vi "Assignment_2_Boolean.vi"() -> ()   [LabVIEW 2019]
uses:
  <vilib>/numeric/Random Number (Range) U64.vi
  <vilib>/numeric/sub_Random U32.vi
panel:
  in  "y":bool
  in  "y":bool
  in  "lower bound (0)":u64
  in  "upper bound (100)":u64=100
  out "Random Number":u64
  out "0, 1":i16
  in  "Boolean":bool
  in  "value 5":dbl
  in  "value 4":dbl
  in  "value 3":dbl
  in  "value 2":dbl
  in  "value 1":dbl
  out "Result":i32
  out "Result":bool
  in  "y":bool
  in  "x":bool
  in  "T/F":bool
  out "Result":bool
  out "Result":bool
  in  "x":bool
  out "Result":bool
  in  "y":bool
  in  "x":bool
  out "Result":bool
  in  "x":bool
  # "Diagram Disabled Structure is used"
  # "And gate/Or gate"
  # "Not And gate/Not Or gate"
  # "Exclusive Or gate/Not Exclusive Or gate"
  # "Not gate"
  # "Implies Operator"
  # "Compond Arithmetic"
  # "Bool to (0, 1)"
  # "Random Number Generator"
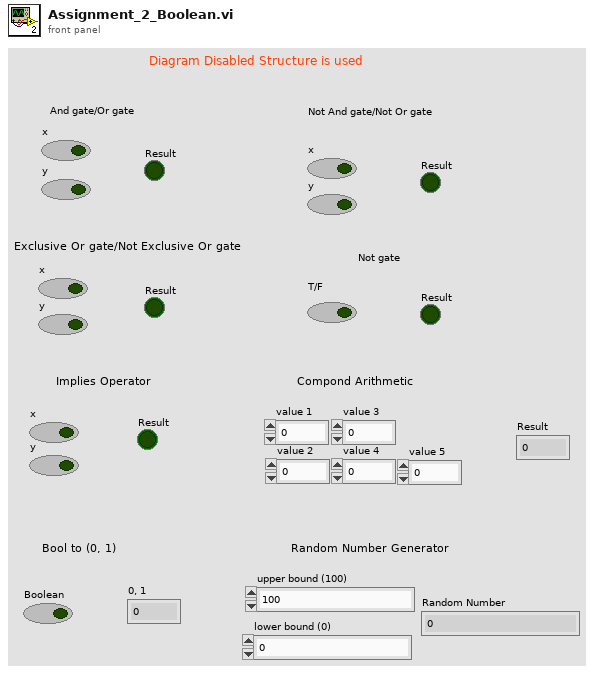
[diagram p1: front panel]
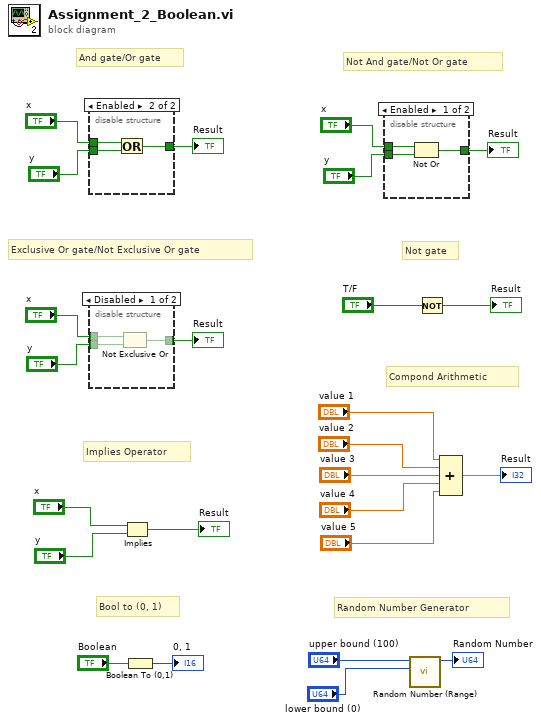
[diagram p0: block diagram]
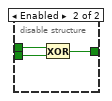
[diagram p2: hidden frame]
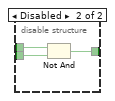
[diagram p3: hidden frame]
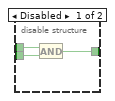
[diagram p4: hidden frame]
diagram:
  # "Random Number Generator"
  # "Bool to (0, 1)"
  # "Compond Arithmetic"
  # "Implies Operator"
  # "Not gate"
  # "Exclusive Or gate/Not Exclusive Or gate"
  # "Not And gate/Not Or gate"
  # "And gate/Or gate"
  n1 = disable-structure shown="Enabled" {
    disable-tunnel: "x" -> [w28 w30]
    disable-tunnel: "y" -> [w27 w29]
    disable-tunnel: [w26 w31] -> w24
    frame Disabled {
      n2 = And(x=w28, y=w27) -> (x .and. y?=w26:bool)
    }
    frame Enabled {
      n3 = Or(x=w30, y=w29) -> (x .or. y?=w31:bool)
    }
  }
  "Result" <- w24
  n4 = disable-structure shown="Disabled" {
    disable-tunnel: "x" -> [w33 w36]
    disable-tunnel: "y" -> [w32 w35]
    disable-tunnel: [w34 w37] -> w19
    frame Disabled {
      n5 = Not Exclusive Or(1:w32, 2:w33) -> (0:w34:bool)
    }
    frame Enabled {
      n6 = Exclusive Or(1:w35, 2:w36) -> (0:w37:bool)
    }
  }
  "Result" <- w19
  n7 = Implies(1:"y", 2:"x") -> (0:→"Result":bool)
  n8 = Boolean To (0,1)(Boolean="Boolean") -> (0, 1=→"0, 1":i16)
  n9 = disable-structure shown="Enabled" {
    disable-tunnel: "x" -> [w39 w42]
    disable-tunnel: "y" -> [w38 w41]
    disable-tunnel: [w40 w43] -> w21
    frame Enabled {
      n10 = Not Or(1:w38, 2:w39) -> (0:w40:bool)
    }
    frame Disabled {
      n11 = Not And(1:w41, 2:w42) -> (0:w43:bool)
    }
  }
  "Result" <- w21
  n12 = call-poly <vilib>:"Random Number (Range).vi"("lower bound (0)"="lower bound (0)", "upper bound (100)"="upper bound (100)") -> ("number"=→"Random Number":u64)  [unwired: 9 in]
  n13 = Not(x="T/F") -> (.not. x?=→"Result":bool)
  n14 = Compound Arithmetic op=ADD("value 1", "value 2", "value 3", "value 4", "value 5") -> (→"Result":dbl)
